vi "Handle Command.vi"(8 "error in":errorcluster, 10 "CMD in":refnum<class "Update Filter State CMD.lvclass">, 11 "Object In":refnum<class>) -> (0 "error out":errorcluster, 1 "Command Successful?":bool, 2 "CMD out":refnum<class "Update Filter State CMD.lvclass">, 3 "Object Out":refnum<class>)   [LabVIEW 2014, in "eCRDS Library.lvlib" / "Update Filter State CMD.lvclass"]
doc: "This VI will contain the code used to actually execute the request. If the request is successful, this will be indicated by the boolean output <b>Command Successful?</b>. The boolean output can then be used by the <b>Command Reply</b> which sends a reply if the reply queue is valid."
uses:
  Update Filter State CMD.lvclass
  reusable/CRDS/Data/Main/CRDS Data.lvclass
  reusable/CRDS/Main/CRDS.lvclass
  reusable/Instrument/Instrument.lvclass/Instrument.ctl
  Update Filter State CMD.lvclass/Update Filter State CMD.ctl
  reusable/Instrument/Read Data.vi
  reusable/Instrument/Read Log Session.vi
  reusable/Instrument/Write Data.vi
  reusable/CRDS/Data/Main/Write filter.vi
  reusable/Data/Data.lvclass
  <userlib>/_Session Fwk/Session - Root.lvclass
  reusable/Session APIs/Session Log/System Log.lvclass
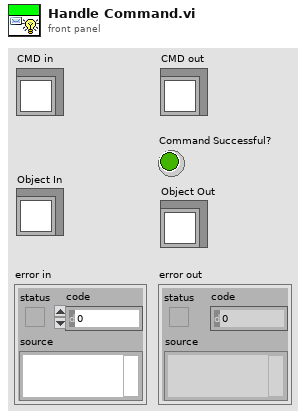
[diagram p1: front panel]
types:
  T1 = typedef "Session - Root.lvclass/Session Handle.ctl" = refnum<data-value>
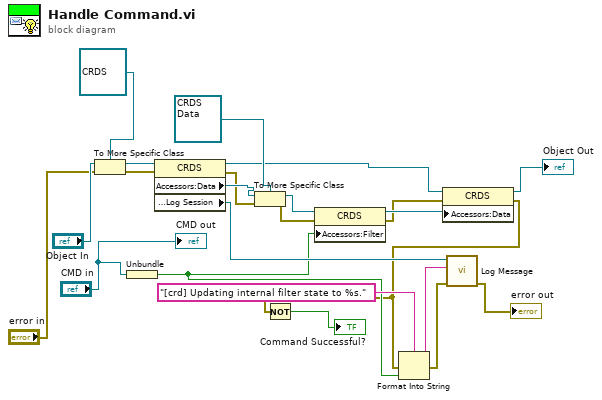
[diagram p0: block diagram]
diagram:
  n1 = To More Specific Class(target class=refnum<class "CRDS.lvclass"> refnum ("CRDS Lib.lvlib:CRDS"), reference="Object In", error in="error in") -> (specific class reference=w22:refnum<class "CRDS.lvclass">, error out=w15:errorcluster)
  n2 = Unbundle("CMD in") -> (w6:bool)
  n3 = property class="CRDS"(reference=w22, error in=w15) -> (reference out=w5:refnum<class "CRDS.lvclass">, error out=w16:errorcluster, "Accessors:Data"=w21:refnum<class "Data.lvclass">, "Accessors:Log Session"=w12:T1)
  n4 = To More Specific Class(target class=refnum<class "CRDS Data.lvclass"> refnum ("CRDS Lib.lvlib:CRDS"), reference=w21, error in=w16) -> (specific class reference=w19:refnum<class "CRDS Data.lvclass">, error out=w17:errorcluster)
  n5 = property class="CRDS"(reference=w19, error in=w17, "Accessors:Filter"=w6) -> (reference out=w3:refnum<class "CRDS Data.lvclass">, error out=w2:errorcluster)
  n6 = property class="CRDS"(reference=w5, error in=w2, "Accessors:Data"=w3) -> (reference out=→"Object Out":refnum<class "CRDS.lvclass">, error out=w1:errorcluster)
  n7 = Not(x=w1) -> (.not. x?=→"Command Successful?":bool)
  n8 = Format Into String(format string="[crd] Updating internal filter state to %s.", error in=w1, w6) -> (resulting string=w9:string, error out=w10:errorcluster)  [unwired: 1 in]
  n9 = call "Log Message.vi"("error in"=w10, "MSG In"=w9, "session in"=w12) -> ("error out"=→"error out":errorcluster)  [unwired: 7 in, 1 out]
  "CMD out" <- "CMD in"
